vi "Get Session Information.vi"(8 "error in (no error)":errorcluster, 11 "Network Interface":refnum<data-value>) -> (0 "error out":errorcluster, 2 "Active Connections":u32, 3 "Network Interface Out":refnum<data-value>)   [LabVIEW 2017]
uses:
  <vilib>/gpm_packages/@cs/Network-sink/Source/Network Interface/Network Interface/Network Interface.lvclass
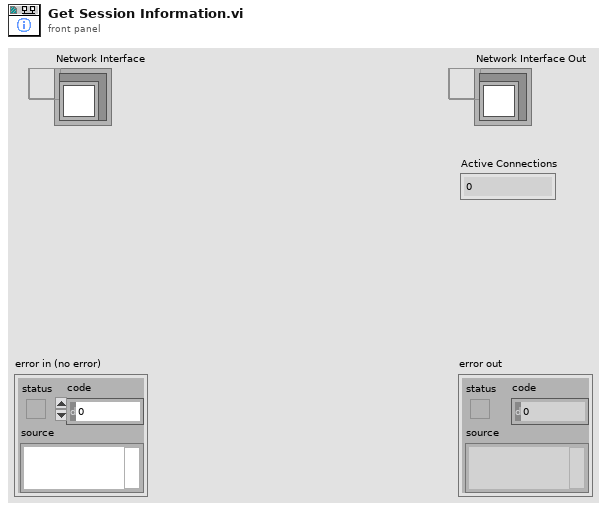
[diagram p1: front panel]
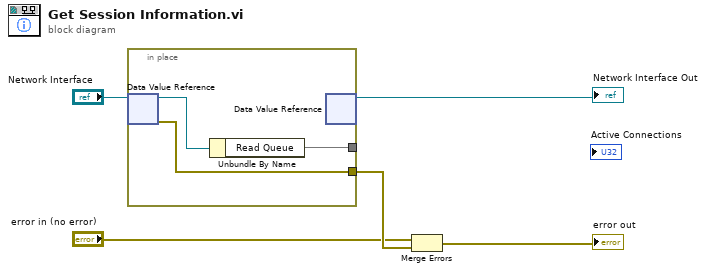
[diagram p0: block diagram]
diagram:
  n1 = in-place {
    in-place-border: [w7] -> _
    in-place-border: [w6] -> w3
    n2 = in-place-dvr #1("Network Interface") -> (w8:refnum<class "Network Interface.lvclass">, w6:errorcluster)
    n3 = Unbundle By Name(w8) -> ("Read Queue"=w7)
    n4 = in-place-dvr #1() -> (→"Network Interface Out":refnum<data-value>)  [unwired: 1 in, 1 out]
  }
  n5 = Merge Errors("error in (no error)", w3) -> (→"error out":errorcluster)
